vi "SaveMotorData.vi"(8 "error in (no error)":errorcluster, 9 "Motor Relative":dbl[](array[numeric]), 11 "Refnum in":refnum<k34>) -> (0 "error out":errorcluster, 3 "Refnum out":refnum<k34>)   [LabVIEW 2018]
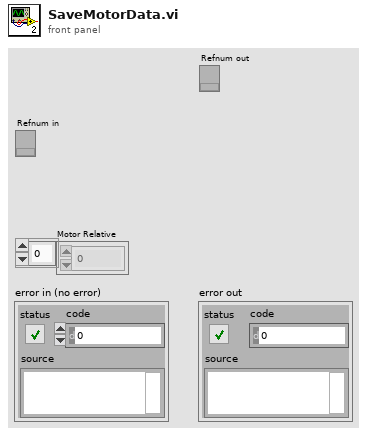
[diagram p1: front panel]
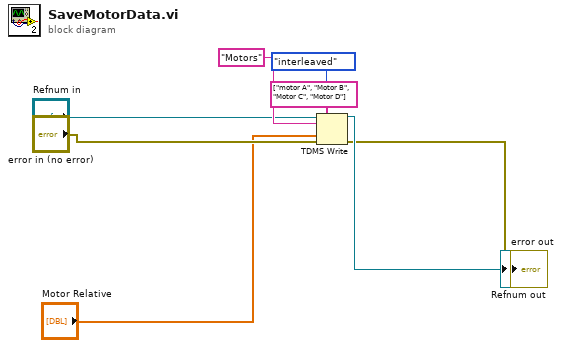
[diagram p0: block diagram]
diagram:
  n1 = TDMS Write(0:"Refnum in", 1:enum16{"decimated", "interleaved"}."interleaved" ("data layout (0:decimated)"), 5:"Motors", 7:string[] ["motor A", "Motor B", "Motor C", "Motor D"] ("channel name(s) in (Untitled)"), 9:"Motor Relative", 11:"error in (no error)") -> (4:→"Refnum out":refnum<k34>, 15:→"error out":errorcluster)  [unwired: 2 out]
